vi "UI Event-Title Bar-Mouse Down.vi"(8 "Error In":errorcluster, 11 "Appearance Actor in":refnum<class "Appearance Actor.lvclass">) -> (0 "Error Out":errorcluster, 3 "Appearance Actor out":refnum<class "Appearance Actor.lvclass">)   [LabVIEW 2021, in "Appearance Actor.lvlib" / "Appearance Actor.lvclass"]
doc: "Handles Mouse Down Event on Title Bar. By Default, call win32 API to move the window. Override this method to change its behavior."
uses:
  Appearance Actor.lvclass
  Appearance Actor.lvclass/Appearance Actor.ctl
  Windows/System32/user32.dll
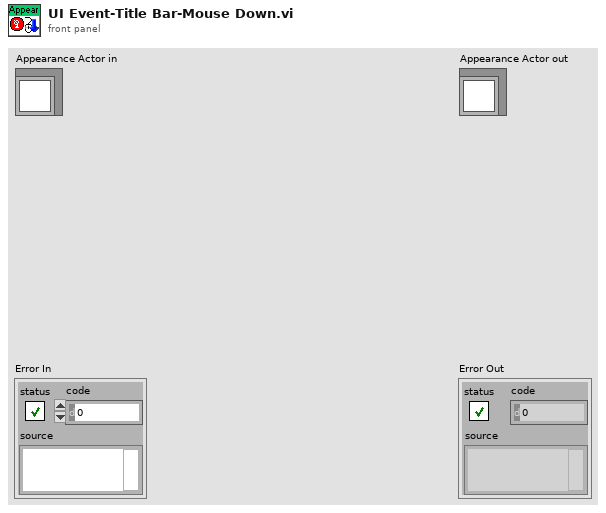
[diagram p1: front panel]
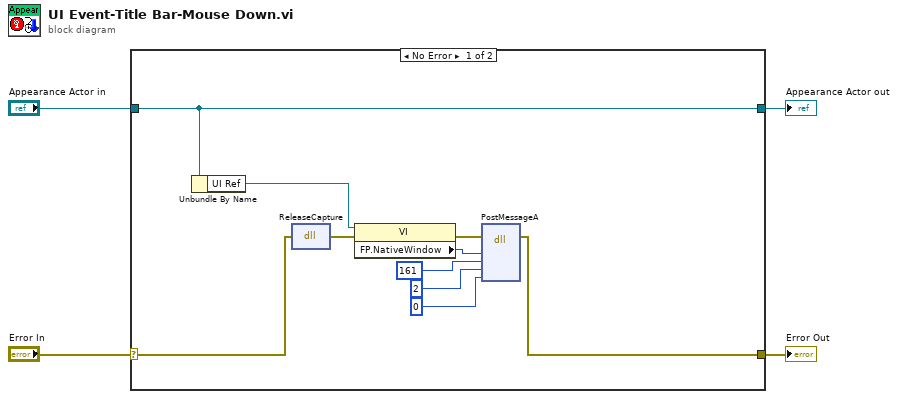
[diagram p0: block diagram]
diagram:
  n1 = case shown="No Error" "Error In" {
    selector: "Error In" -> [w9 w16]
    tunnel: [w8 w16] -> w3
    tunnel: [w6 w15] -> w1
    tunnel: "Appearance Actor in" -> [w6 w15]
    frame No Error {
      n2 = Unbundle By Name(w6) -> ("UI Ref"=w5:refnum<vi>)
      n3 = dll-call lib="C:/Windows/System32/user32.dll" fn="ReleaseCapture"(error in=w9) -> (error out=w14:errorcluster)  [unwired: 3 in, 1 out]
      n4 = property class="VI"(reference=w5, error in=w14) -> (error out=w7:errorcluster, "FP.NativeWindow"=w13:u64)  [unwired: 1 out]
      n5 = dll-call lib="C:/Windows/System32/user32.dll" fn="PostMessageA"(error in=w7, "arg1"=w13, "arg2"=161, "arg3"=2, "arg4"=0) -> (error out=w8:errorcluster)  [unwired: 7 in, 1 out]
    }
    frame Error {
    }
  }
  "Error Out" <- w3
  "Appearance Actor out" <- w1
